vi "Merge into Error.vi"(2 "Boolean in":bool, 3 "error in (no error)":errorcluster) -> (7 "Boolean out":bool)   [LabVIEW 2017]
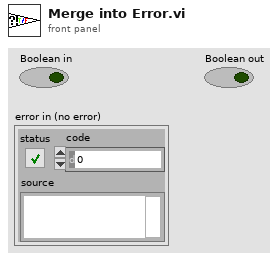
[diagram p1: front panel]
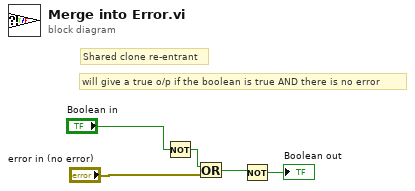
[diagram p0: block diagram]
diagram:
  # "Shared clone re-entrant"
  # "will give a true o/p if the boolean is true AND there is no error"
  n1 = Not(x="Boolean in") -> (.not. x?=w3:bool)
  n2 = Or(x=w3, y="error in (no error)") -> (x .or. y?=w1:bool)
  n3 = Not(x=w1) -> (.not. x?=→"Boolean out":bool)
